vi "userauth_hostbased_fromfile.vi"() -> ()   [LabVIEW 2017]
doc: "Illustrates how to authenticate a session using public key, read from file."
uses:
  libssh2/libssh2_session_handshake_tcp.vi
  libssh2/libssh2_init_default.vi
  libssh2/libssh2_session_init_ex.vi
  <vilib>/Utility/tcp.llb/TCP Get Raw Net Object.vi
  libssh2/libssh2_session_handshake_socket.vi
  libssh2/libssh2.lvlib
panel:
  in  "local_username":string
  in  "local_hostname":string
  out "authenticated":bool
  in  "private key":path
  in  "public key":path
  in  "passphrase":string
  in  "username":string
  in  "hostname":string="localhost"
  out "error out":errorcluster
  # "This is the public key file (e.g., generated with ssh-keygen)"
  # "This is the private key file (e.g., generated with ssh-keygen)\n\nImportant: If your key files don't work, try generating keys\nwith the following command: \"ssh-keygen -m PEM -t rsa\".\nThis will create a key file with the header\n\"-----BEGIN RSA PRIVATE KEY-----\" as is expected by libssh2."
  # "This is the passphrase for your private key."
  # "When everything goes right, this status should be TRUE."
  # "Important\nThis only works when libssh2 is backed by OpenSSL. You can verify the crypo-library of your version\nof libssh2 with libssh2_crypto_engine.vi"
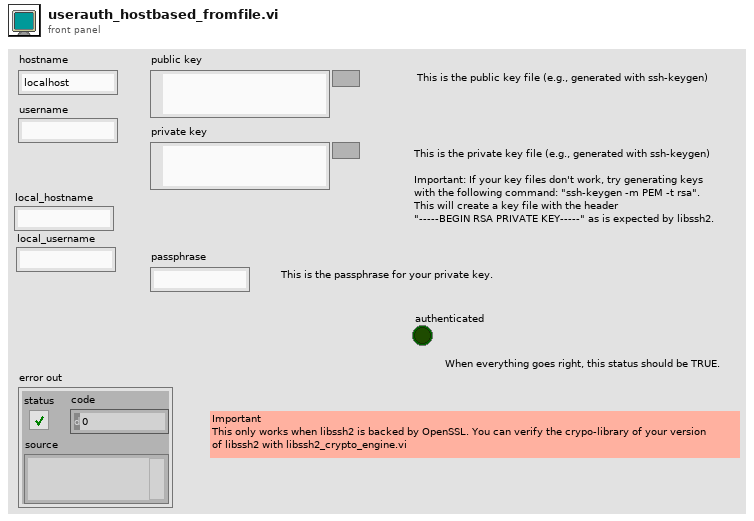
[diagram p1: front panel]
types:
  T1 = typedef "libssh2.lvlib/Session Refnum.ctl" = refnum<k1>
  T2 = typedef "libssh2.lvlib/libssh2_crypto_engine.ctl" = enum16{"no crypto", "OpenSSL", "gcrypt", "mbedTLS", "WinCNG", "OS400qc3"}
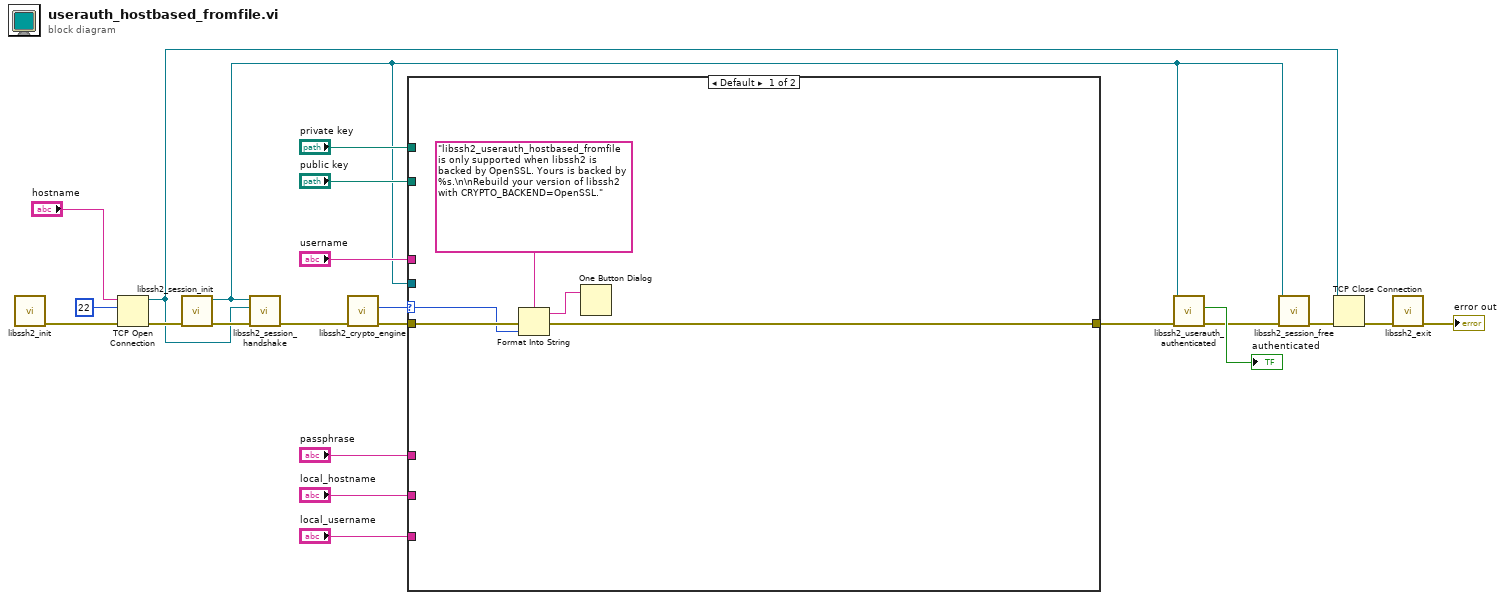
[diagram p0: block diagram]
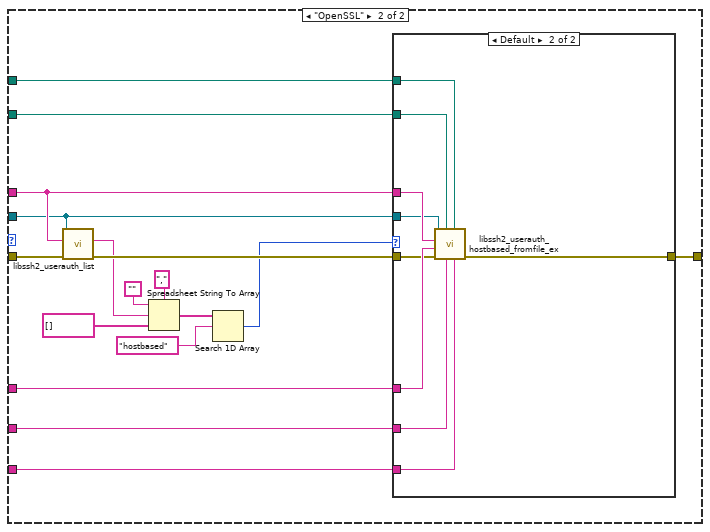
[diagram p2: hidden frame]
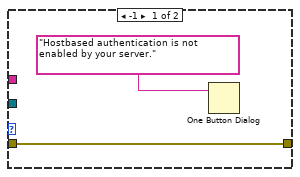
[diagram p3: hidden frame]
diagram:
  n1 = call-poly "libssh2_init.vi"() -> ("error out"=w22:errorcluster)  [unwired: 11 in]
  n2 = TCP Open Connection(address="hostname", remote port or service name=u16 22, error in (no error)=w22) -> (connection ID=w14:refnum<k5>, error out=w15:errorcluster)  [unwired: 2 in]
  n3 = call "libssh2_session_init.vi"("error in (no error)"=w15) -> ("error out"=w17:errorcluster, "session"=w1:T1)  [unwired: 9 in]
  n4 = call-poly "libssh2_session_handshake.vi"("error in (no error)"=w17, "tcp connection"=w14, "session"=w1) -> ("error out"=w4:errorcluster)  [unwired: 8 in]
  n5 = call "libssh2_crypto_engine.vi"("error in (no error)"=w4) -> ("error out"=w3:errorcluster, "crypto engine"=w2:T2)  [unwired: 9 in]
  n6 = case shown="Default" w2 {
    selector: w2 -> [w23 _]
    tunnel: [w24 w44] -> w13
    tunnel: "passphrase" -> [_ w43]
    tunnel: "public key" -> [_ w42]
    tunnel: "private key" -> [_ w41]
    tunnel: "local_hostname" -> [_ w40]
    tunnel: "local_username" -> [_ w39]
    tunnel: w3 -> [w25 w38]
    tunnel: "username" -> [_ w36]
    tunnel: w1 -> [_ w28]
    frame Default {
      n7 = Format Into String(format string="libssh2_userauth_hostbased_fromfile is only supported when libssh2 is backed by OpenSSL. Yours is backed by %s.\n\nRebuild your version of libssh2 with CRYPTO_BACKEND=OpenSSL.", error in=w25, w23) -> (resulting string=w26:string, error out=w24:errorcluster)  [unwired: 1 in]
      n8 = One Button Dialog(message=w26) -> ()  [unwired: 1 in, 1 out]
    }
    frame "OpenSSL" {
      n9 = call "libssh2_userauth_list.vi"("error in (no error)"=w38, "username"=w36, "session"=w28) -> ("error out"=w37:errorcluster, "supported authentication schemes"=w35:string)  [unwired: 7 in]
      n10 = Spreadsheet String To Array(delimiter (Tab)=",", format string="", spreadsheet string=w35, array type (2D Dbl)=string[] []) -> (array=w31:string[])
      n11 = Search 1D Array(1D array=w31, element="hostbased") -> (index of element=w29:i32)  [unwired: 1 in]
      n12 = case shown="Default" w29 {
        tunnel: [w46 w55] -> w44
        tunnel: w43 -> [_ w54]
        tunnel: w42 -> [_ w53]
        tunnel: w41 -> [_ w52]
        tunnel: w40 -> [_ w51]
        tunnel: w39 -> [_ w50]
        tunnel: w37 -> [w46 w49]
        tunnel: w36 -> [_ w48]
        tunnel: w28 -> [_ w47]
        frame -1 {
          n13 = One Button Dialog(message="Hostbased authentication is not enabled by your server.") -> ()  [unwired: 1 in, 1 out]
        }
        frame Default {
          n14 = call "libssh2_userauth_hostbased_fromfile_ex.vi"("local_username"=w50, "private key"=w52, "hostname"=w51, "public key"=w53, "error in (no error)"=w49, "passphrase"=w54, "username"=w48, "session"=w47) -> ("error out"=w55:errorcluster)  [unwired: 3 in]
        }
      }
    }
  }
  n15 = call "libssh2_userauth_authenticated.vi"("error in (no error)"=w13, "session"=w1) -> ("error out"=w8:errorcluster, "authenticated"=→"authenticated":bool)  [unwired: 8 in]
  n16 = call "libssh2_session_free.vi"("error in (no error)"=w8, "session"=w1) -> ("error out"=w16:errorcluster)  [unwired: 9 in]
  n17 = TCP Close Connection(connection ID=w14, error in (no error)=w16) -> (error out=w19:errorcluster)  [unwired: 1 in, 1 out]
  n18 = call "libssh2_exit.vi"("error in (no error)"=w19) -> ("error out"=→"error out":errorcluster)  [unwired: 10 in]
